vi "Insert data into array.vi"(4 "Bin width (pixels)":dbl, 5 "current snapshot number":dbl, 6 "End wavelength of raster scan":dbl[unit], 7 "To Append":T1, 8 "Start wavelength of raster scan":dbl[unit], 9 "Bins per scan":dbl, 10 "Bin width (nm)":dbl[unit], 11 "Main data array for raster scan, before this this snapshot":cluster{dbl[unit], dbl[]}[](array[cluster])) -> (1 "new version of Emma and John Data Array for current snapshot":i32[](array[numeric]), 2 "Emma and John Data Array for current snapshot":i32[](array[numeric]), 3 "Main data array for raster scan,\nas modified after this snapshot":cluster{dbl[unit], dbl[]}[](array[cluster]))   [LabVIEW 2017, in "Synapse CCD.lvclass"]
uses:
  Synapse CCD.lvclass
  <vilib>/Analysis/baseanly.llb/Mean (DBL).vi
  <vilib>/Analysis/NI_AALBase.lvlib
panel:
  out "Numeric":dbl[unit]
  out "Array of Wavelengths":dbl[](array[numeric])
  out "left edge of active area":dbl[unit]
  out "right edge of active area":dbl[unit]
  out "Emma and John kept points wavelength array":dbl[](array[numeric])
  out "Bin center wavelength":dbl[unit]
  out "Bin center wavelength 2":dbl[unit]
  in  "Total Pixels":dbl=1024.0
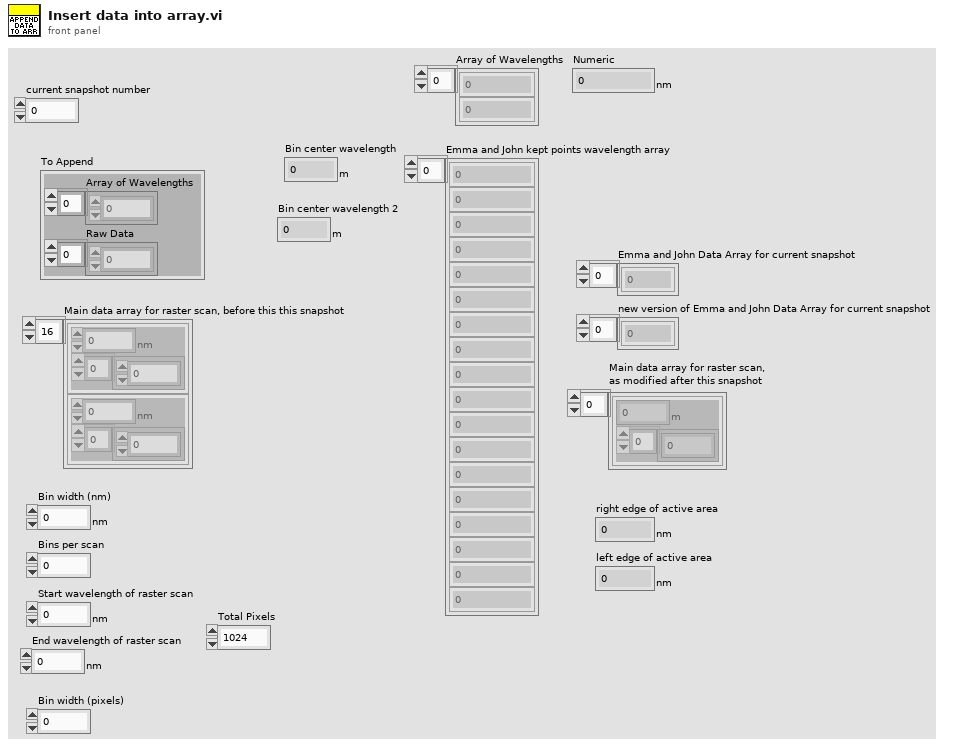
[diagram p1: front panel]
types:
  T1 = cluster{"Array of Wavelengths":dbl[], "Raw Data":i32[]}
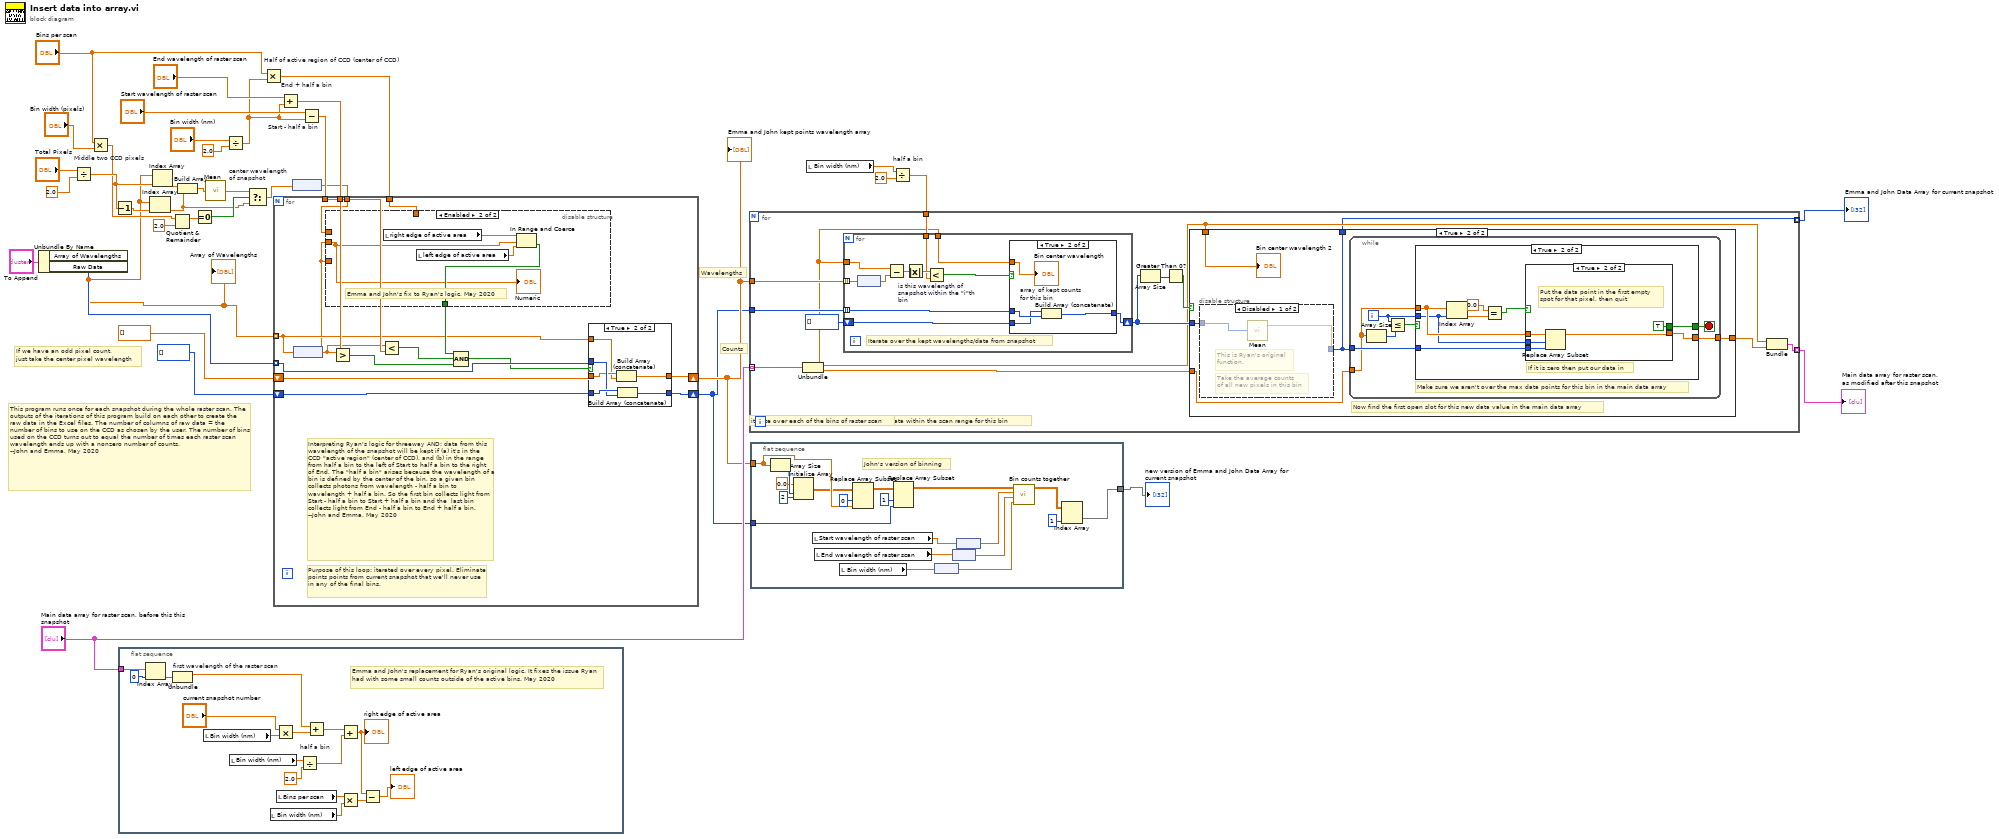
[diagram p0: block diagram]
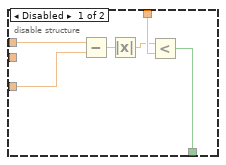
[diagram p2: hidden frame]
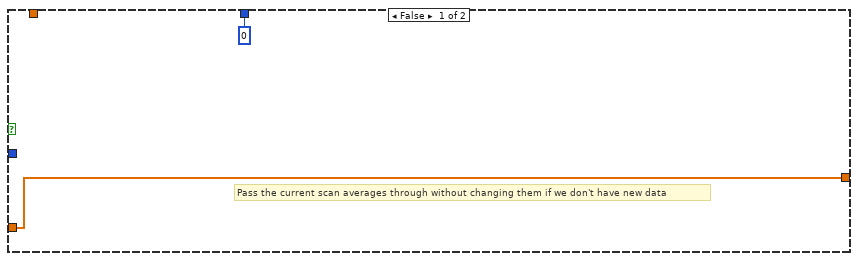
[diagram p4: hidden frame]
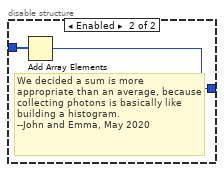
[diagram p5: hidden frame]
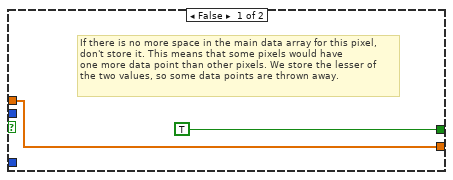
[diagram p6: hidden frame]
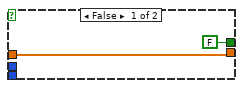
[diagram p7: hidden frame]
diagram:
  # "This program runs once for each snapshot during the whole raster scan. The outputs of the iterations of this program build on each other to create the raw data in the Excel files. The number of columns of raw data = the number of bins to use on the CCD as chosen by the user. The number of bins used on the CCD turns out to equal the number of times each raster scan wavelength ends up with a nonzero number of counts.\n--John and Emma, May 2020"
  # "If we have an odd pixel count, \njust take the center pixel wavelength"
  # "Counts"
  # "Wavelengths"
  n1 = Unbundle By Name("To Append") -> ("Array of Wavelengths"=w4:dbl[], "Raw Data"=w37:i32[])
  "Array of Wavelengths" <- w4
  n2 = Divide "Middle two CCD pixels"(x="Total Pixels", y=2.0) -> (x/y=w22:dbl)
  n3 = Multiply(x="Bins per scan", y="Bin width (pixels)") -> (x*y=w12:dbl)
  n4 = Decrement(x=w22) -> (x-1=w21:dbl)
  n5 = flat-sequence {
    tunnel: "Main data array for raster scan, before this this snapshot" -> [w54]
    frame #0 {
      # "Emma and John's replacement for Ryan's original logic. It fixes the issue Ryan had with some small counts outside of the active bins. May 2020"
      n6 = Index Array(array=w54, index=0) -> (element=w53:cluster{dbl[unit], dbl[]})
      n7 = Unbundle "first wavelength of the raster scan"(w53) -> (w43:dbl[unit])  [unwired: 1 out]
      n8 = local read "Bin width (nm)"() -> (w41:dbl[unit])
      n9 = local read "Bin width (nm)"() -> (w52:dbl[unit])
      n10 = local read "Bin width (nm)"() -> (w48:dbl[unit])
      n11 = Multiply(x="current snapshot number", y=w41) -> (x*y=w42:dbl[unit])
      n12 = local read "Bins per scan"() -> (w49:dbl)
      n13 = Divide "half a bin"(x=w52, y=2.0) -> (x/y=w50:dbl[unit])
      n14 = Add(x=w43, y=w42) -> (x+y=w39:dbl[unit])
      n15 = Add(x=w39, y=w50) -> (x+y=w47:dbl[unit])
      "right edge of active area" <- w47
      n16 = Multiply(x=w49, y=w48) -> (x*y=w46:dbl[unit])
      n17 = Subtract(x=w47, y=w46) -> (x-y=→"left edge of active area":dbl[unit])
    }
  }
  n18 = Index Array(array=w4, index=w21) -> (element=w8:dbl)
  n19 = Index Array(array=w4, index=w22) -> (element=w20:dbl)
  n20 = Quotient & Remainder(x=w12, y=2.0) -> (x-y*floor(x/y)=w11:dbl)  [unwired: 1 out]
  n21 = Build Array(w20, w8) -> (w19:dbl[])
  n22 = Equal To 0?(x=w11) -> (x = 0?=w10:bool)
  n23 = call-poly <vilib>:"Mean.vi"("X"=w19) -> ("mean"=w9:dbl)  [unwired: 1 out]
  n24 = Divide(x="Bin width (nm)", y=2.0) -> (x/y=w18:dbl[unit])
  n25 = Select "center wavelength\nof snapshot"(t=w9, s=w10, f=w8) -> (s? t:f=w7:dbl)
  n26 = Multiply "Half of active region of CCD (center of CCD)"(x="Bins per scan", y=w18) -> (x*y=w16:dbl[unit])
  n27 = Add "End + half a bin"(x="End wavelength of raster scan", y=w18) -> (x+y=w31:dbl[unit])
  n28 = node(w7) -> (w17:dbl[unit])
  n29 = Subtract "Start - half a bin"(x="Start wavelength of raster scan", y=w18) -> (x-y=w36:dbl[unit])
  n30 = for {
    tunnel: w4 -> [w56] mode=indexing
    tunnel: w37 -> [w69] mode=indexing
    shift-right: [w65] -> w2
    shift-left: i32[] [] ("appended array") -> [w68]
    shift-right: [w66] -> w3
    shift-left: dbl[] [] ("appended array") -> [w67]
    tunnel: w31 -> [w64]
    tunnel: w36 -> [w63]
    tunnel: w17 -> [w62]
    tunnel: w16 -> [w61]
    # "Purpose of this loop: iterated over every pixel. Eliminate points points from current snapshot that we'll never use in any of the final bins."
    # "Interpreting Ryan's logic for threeway AND: data from this wavelength of the snapshot will be kept if (a) it's in the CCD \"active region\" (center of CCD), and (b) in the range from half a bin to the left of Start to half a bin to the right of End. The \"half a bin\" arises because the wavelength of a bin is defined by the center of the bin, so a given bin collects photons from wavelength - half a bin to  wavelength + half a bin. So the first bin collects light from Start - half a bin to Start + half a bin and the  last bin collects light from End - half a bin to End + half a bin.\n--John and Emma, May 2020"
    n31 = node(w56) -> (w55:dbl[unit])
    n32 = disable-structure shown="Enabled" {
      disable-tunnel: w62 -> [w75 _]
      disable-tunnel: w61 -> [w74 _]
      disable-tunnel: w55 -> [w72 _]
      disable-tunnel: [w70 w79] -> w59
      disable-tunnel: w55 -> [_ w78]
      frame Disabled {
        n33 = Subtract(x=w75, y=w72) -> (x-y=w73:dbl[unit])
        n34 = Absolute Value(x=w73) -> (abs(x)=w71:dbl[unit])
        n35 = Less?(x=w71, y=w74) -> (x < y?=w70:bool)
      }
      frame Enabled {
        # "Emma and John's fix to Ryan's logic, May 2020"
        n36 = local read "right edge of active area"() -> (w76:dbl[unit])
        n37 = local read "left edge of active area"() -> (w77:dbl[unit])
        n38 = In Range and Coerce(upper limit=w76, x=w78, lower limit=w77) -> (In Range?=w79:bool)  [unwired: 1 out]
        "Numeric" <- w78
      }
    }
    n39 = Greater?(x=w55, y=w63) -> (0:w58:bool)
    n40 = Less?(x=w55, y=w64) -> (x < y?=w57:bool)
    n41 = Compound Arithmetic op=AND(w59, w57, w58) -> (w60:bool)
    n42 = case shown="True" w60 {
      tunnel: w56 -> [_ w82]
      tunnel: w69 -> [_ w84]
      tunnel: w68 -> [w80 w85]
      tunnel: w67 -> [w81 w83]
      tunnel: [w81 w87] -> w66
      tunnel: [w80 w86] -> w65
      frame False {
      }
      frame True {
        n43 = Build Array (concatenate)(w83, w82) -> (w87:dbl[])
        n44 = Build Array (concatenate)(w85, w84) -> (w86:i32[])
      }
    }
  }
  "Emma and John kept points wavelength array" <- w3
  n45 = flat-sequence {
    tunnel: w3 -> [w103]
    tunnel: w2 -> [w98]
    tunnel: [w88] -> w1
    frame #0 {
      # "John's version of binning"
      n46 = Array Size(array=w103) -> (size(s)=w105:i32)
      n47 = Initialize Array(0.0 ("element"), w105, 2 ("dimension size")) -> (w102:dbl[][])
      n48 = local read "Start wavelength of raster scan"() -> (w96:dbl[unit])
      n49 = local read "End wavelength of raster scan"() -> (w95:dbl[unit])
      n50 = local read "Bin width (nm)"() -> (w94:dbl[unit])
      n51 = Replace Array Subset(array=w102, new element=w103, index (col)=0 ("disabled index (col)")) -> (w99:dbl[][])  [unwired: 1 in]
      n52 = Replace Array Subset(array=w99, new element=w98, index (col)=1) -> (w97:dbl[][])  [unwired: 1 in]
      n53 = node(w94) -> (w91:dbl)
      n54 = node(w95) -> (w92:dbl)
      n55 = node(w96) -> (w93:dbl)
      n56 = call "Bin counts together.vi"("bin width (unitless, assumed nm)"=w91, "center wavelength \nof last bin  (unitless, assumed nm)"=w92, "center wavelength \nof first bin (unitless, assumed nm)"=w93, "Array of wavelengths \nand counts (unitless, assumed nm)"=w97) -> ("binned array of wavelengths \nand counts (unitless, assumed nm)"=w90:dbl[][])  [unwired: 7 in]
      n57 = Index Array(array=w90, index (col)=1 ("disabled index (col)")) -> (element=w88:dbl[])  [unwired: 1 in]
    }
  }
  n58 = local read "Bin width (nm)"() -> (w27:dbl[unit])
  n59 = Divide "half a bin"(x=w27, y=2.0) -> (x/y=w26:dbl[unit])
  n60 = for {
    tunnel: "Main data array for raster scan, before this this snapshot" -> [w119] mode=indexing
    tunnel: w3 -> [w118]
    tunnel: w2 -> [w117]
    tunnel: w26 -> [w116]
    tunnel: [w113] -> w25 mode=indexing
    tunnel: [w107] -> w6 mode=indexing
    # "iterate over each of the bins of raster scan"
    # "Only try to add a new count if we have new data within the scan range for this bin"
    n61 = Unbundle(w119) -> (w108:dbl[unit], w115:dbl[])
    n62 = for {
      tunnel: w108 -> [w165]
      tunnel: w118 -> [w163] mode=indexing
      tunnel: w117 -> [w158] mode=indexing
      tunnel: w116 -> [w160]
      shift-right: [w157] -> w109
      shift-left: i32[] [] -> [w156]
      tunnel: w108 -> [w155]
      # "Iterate over the kept wavelengths/data from snapshot"
      n63 = node(w163) -> (w162:dbl[unit])
      n64 = Subtract(x=w165, y=w162) -> (x-y=w164:dbl[unit])
      n65 = Absolute Value(x=w164) -> (abs(x)=w161:dbl[unit])
      n66 = Less? "is this wavelength of snapshot within the \"i\"th bin"(x=w161, y=w160) -> (x < y?=w159:bool)
      n67 = case shown="True" w159 {
        tunnel: w158 -> [_ w168]
        tunnel: [w166 w170] -> w157
        tunnel: w156 -> [w166 w167]
        tunnel: w155 -> [_ w169]
        frame False {
        }
        frame True {
          n68 = Build Array (concatenate) "array of kept counts \nfor this bin"(w167, w168) -> (w170:i32[])
          "Bin center wavelength" <- w169
        }
      }
    }
    n69 = Array Size(array=w109) -> (size(s)=w111:i32)
    n70 = Greater Than 0?(x=w111) -> (x > 0?=w110:bool)
    n71 = case shown="True" w110 {
      tunnel: w115 -> [w121 w126]
      tunnel: [w121 w125] -> w114
      tunnel: w109 -> [_ w123]
      tunnel: w108 -> [_ w124]
      tunnel: [0 w122] -> w107
      frame False {
        # "Pass the current scan averages through without changing them if we don't have new data"
      }
      frame True {
        # "Now find the first open slot for this new data value in the main data array"
        n72 = disable-structure shown="Disabled" {
          disable-tunnel: [w128 w129] -> w122
          disable-tunnel: w123 -> [w127 w130]
          frame Disabled {
            # "Take the average counts \nof all new pixels in this bin"
            # "This is Ryan's original \nfunction."
            n73 = call-poly <vilib>:"Mean.vi"("X"=w127) -> ("mean"=w128:dbl)  [unwired: 1 out]
          }
          frame Enabled {
            # "We decided a sum is more appropriate than an average, because collecting photons is basically like building a histogram. \n--John and Emma, May 2020"
            n74 = Add Array Elements(numeric array=w130) -> (sum=w129:i32)
          }
        }
        n75 = while {
          tunnel: w126 -> [w131]
          tunnel: w122 -> [w134]
          tunnel: [w133] -> w125
          i -> [w137]
          stop <- w135 stop-if-true
          # "Make sure we aren't over the max data points for this bin in the main data array"
          n76 = Array Size(array=w131) -> (size(s)=w132:i32)
          n77 = Less Or Equal?(x=w137, y=w132) -> (x <= y?=w136:bool)
          n78 = case shown="True" w136 {
            tunnel: w131 -> [w138 w144]
            tunnel: w137 -> [_ w143]
            tunnel: [TRUE w141] -> w135
            tunnel: w134 -> [_ w142]
            tunnel: [w138 w140] -> w133
            frame False {
              # "If there is no more space in the main data array for this pixel,\ndon't store it. This means that some pixels would have \none more data point than other pixels. We store the lesser of\nthe two values, so some data points are thrown away."
            }
            frame True {
              # "If it is zero then put our data in"
              n79 = Index Array(array=w144, index=w143) -> (element=w147:dbl)
              n80 = Equal?(x=0.0, y=w147) -> (x = y?=w145:bool)
              n81 = case shown="True" w145 {
                tunnel: w144 -> [w149 w154]
                tunnel: w143 -> [_ w153]
                tunnel: w142 -> [_ w152]
                tunnel: [w149 w151] -> w140
                tunnel: [FALSE TRUE] -> w141
                frame False {
                }
                frame True {
                  # "Put the data point in the first empty\nspot for that pixel, then quit"
                  n82 = Replace Array Subset(array=w154, new element=w152, index=w153) -> (w151:dbl[])
                }
              }
            }
          }
        }
        "Bin center wavelength 2" <- w124
      }
    }
    n83 = Bundle(w108, w114) -> (w113:cluster{dbl[unit], dbl[]})  [unwired: 1 in]
  }
  "Main data array for raster scan,\nas modified after this snapshot" <- w25
  "Emma and John Data Array for current snapshot" <- w6
  "new version of Emma and John Data Array for current snapshot" <- w1
